vi "number1_sub1-configure data acquisition.vi"(5 "OK Button":bool) -> (1 "samples per acquisition 2":dbl, 2 "sampling rate (samples/sec) 2":dbl)   [LabVIEW 2014]
panel:
  in  "samples per acquisition":dbl=10000.0
  in  "sampling rate (samples/sec)":dbl=1000.0
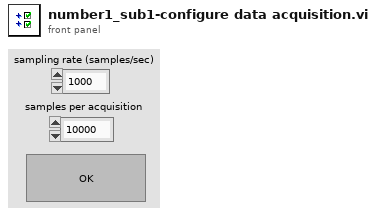
[diagram p1: front panel]
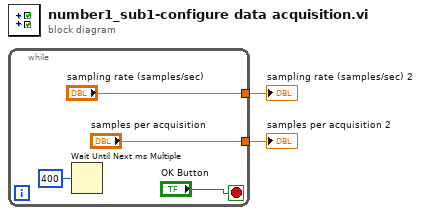
[diagram p0: block diagram]
diagram:
  n1 = while {
    tunnel: ["sampling rate (samples/sec)"] -> w1
    tunnel: ["samples per acquisition"] -> w2
    stop <- "OK Button" stop-if-true
    n2 = Wait Until Next ms Multiple(millisecond multiple=u32 400) -> ()  [unwired: 1 out]
  }
  "samples per acquisition 2" <- w2
  "sampling rate (samples/sec) 2" <- w1
